vi "Main.vi"(7 "IP-Address":string, 11 "Module Admin":refnum<class "Delacor_lib_QMH_Module Admin.lvclass">) -> ()   [LabVIEW 2021, in "Safety.lvlib"]
doc: "This template is based off of the Queued Message Handler design pattern and the Queued Message Handler project template that ships with LabVIEW.\n\nThe main difference is that the queue is private to this module and communication between modules is performed via Broadcast and Request events.\n\nRequest events are wrapped in public API methods and are handled in the Event Handling Loop (EHL) of this VI. Any module can register for Broadcast events sent by this module. The EHL generates messages based on user interface actions.\n\nThe Message Handling Loop (MHL) processes messages generated by the EHL, or by other messages. The messages are string values, so new messages can be added easily to the Message Cases case structure in the MHL. Each message cluster can also provide an optional value for Message Data, which is a variant that can be converted to whatever message-specific data is required.\n_____\nBased on DQMH Project Template 7.0.1.1316."
uses:
  Safety.lvlib
  <vilib>/Delacor/Delacor QMH/Libraries/Module Admin_class/Delacor_lib_QMH_Module Admin.lvclass
  Module Data--cluster.ctl
  <vilib>/Wovalab/Utilities/Helper Loop Periodic Timing/Helper Loop Periodic Timing.lvclass/Helper Loop Periodic Timing.ctl
  <vilib>/Delacor/Delacor QMH/Libraries/Message Queue_class/Delacor_lib_QMH_Message Queue.lvclass/Delacor_lib_QMH_Message Queue.ctl
  Do Something Argument--cluster.ctl
  Do Something Else Argument--cluster.ctl
  Do Something Else and Wait for Reply Argument--cluster.ctl
  Do Something Else and Wait (Reply Payload)--cluster.ctl
  Stop Argument--cluster.ctl
  <vilib>/Delacor/Delacor QMH/Libraries/Module Admin_class/Delacor_lib_QMH_Module Admin.lvclass/Delacor_lib_QMH_Module Admin.ctl
  <vilib>/Utility/miscctls.llb/LVPointTypeDef.ctl
  <vilib>/Delacor/Delacor QMH/Libraries/Message Queue_class/Delacor_lib_QMH_Enqueue Message (Single).vi
  <vilib>/Delacor/Delacor QMH/Libraries/Module Admin_class/Delacor_lib_QMH_Get External Launch.vi
  <vilib>/Wovalab/Utilities/Helper Loop Periodic Timing/U32 Max Value--constant.vi
  <vilib>/Wovalab/Utilities/Helper Loop Periodic Timing/Update Last Execution Time.vi
  <vilib>/Wovalab/Utilities/Helper Loop Periodic Timing/Helper Loop Periodic Timing.lvclass
  <vilib>/Delacor/Delacor QMH/Libraries/Message Queue_class/Delacor_lib_QMH_Message Queue.lvclass
  <userlib>/_OpenG.lib/time/time.llb/openg_time.lvlib
panel:
  out "error out":errorcluster
  out "X":dbl
  out "Status":string
  in  "Simulate MHL Error":bool
  in  "Simulate EHL Error":bool
  in  "Do Something Else <Replace Me>":bool
  in  "Do Something <Replace Me>":bool
  # "These controls have associated \"Value Changed\" events configured in the Event Structure on the diagram.\n\nReplace them (and reconfigure the Event Structure) with the controls you need for your application. \n\nOther processes communicate with this Module via its Public API (wrappers for its Request Events).\n\nThis Module communicates with other processes via its Broadcast Events.\nAny process that wants to receive these messages can register for this module's Broadcast events."
  # "This template is for the DQMH framework. See the block diagram for more information on how to use this template."
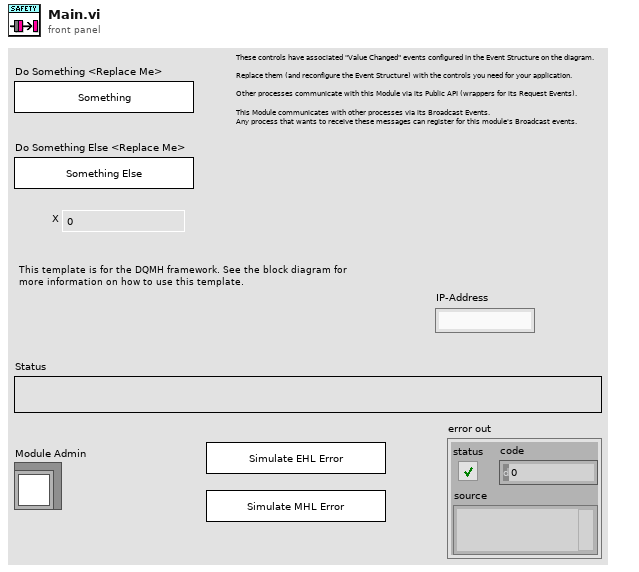
[diagram p1: front panel]
types:
  T1 = typedef "Safety.lvlib/Request Events--cluster.ctl" = cluster{"Stop Module":refnum<user-event>, "Do Something":refnum<user-event>, "Do Something Else":refnum<user-event>, "Do Something Else and Wait for Reply":refnum<user-event>, "Show Panel":refnum<user-event>, "Hide Panel":refnum<user-event>, "Get Module Execution Status":refnum<user-event>, "Show Diagram":refnum<user-event>}
  T2 = typedef "Safety.lvlib/Module Data--cluster.ctl" = cluster{"Status":string, "IP-Address":string}
  T3 = typedef "Safety.lvlib/Do Something Argument--cluster.ctl" = cluster{"Do Something Msg":string}
  T4 = typedef "Safety.lvlib/Do Something Else Argument--cluster.ctl" = cluster{"Do Something Else Msg":string, "X":dbl}
  T5 = typedef "Safety.lvlib/Do Something Else and Wait for Reply Argument--cluster.ctl" = cluster{"Do Something Else Msg":string, "X":dbl, "Wait Notifier":refnum<notifier>, "wait for reply":bool}
  T6 = enum32{"invalid lock state", "Not Locked", "Locked (No Password)", "Password-protected"}
  T7 = typedef "Safety.lvlib/Stop Argument--cluster.ctl" = cluster{"Origin":string, "Exit via Stop Module Req?":bool, "Wait for Module to stop?":bool}
  T8 = typedef "LVPointTypeDef.ctl" = cluster{"Horizontal":i16, "Vertical":i16}
  T9 = enum32{"Invalid", "Standard", "Closed", "Hidden", "Minimized", "Maximized"}
  T10 = typedef "Safety.lvlib/Do Something Else and Wait (Reply Payload)--cluster.ctl" = cluster{"Value":dbl, "error":errorcluster}
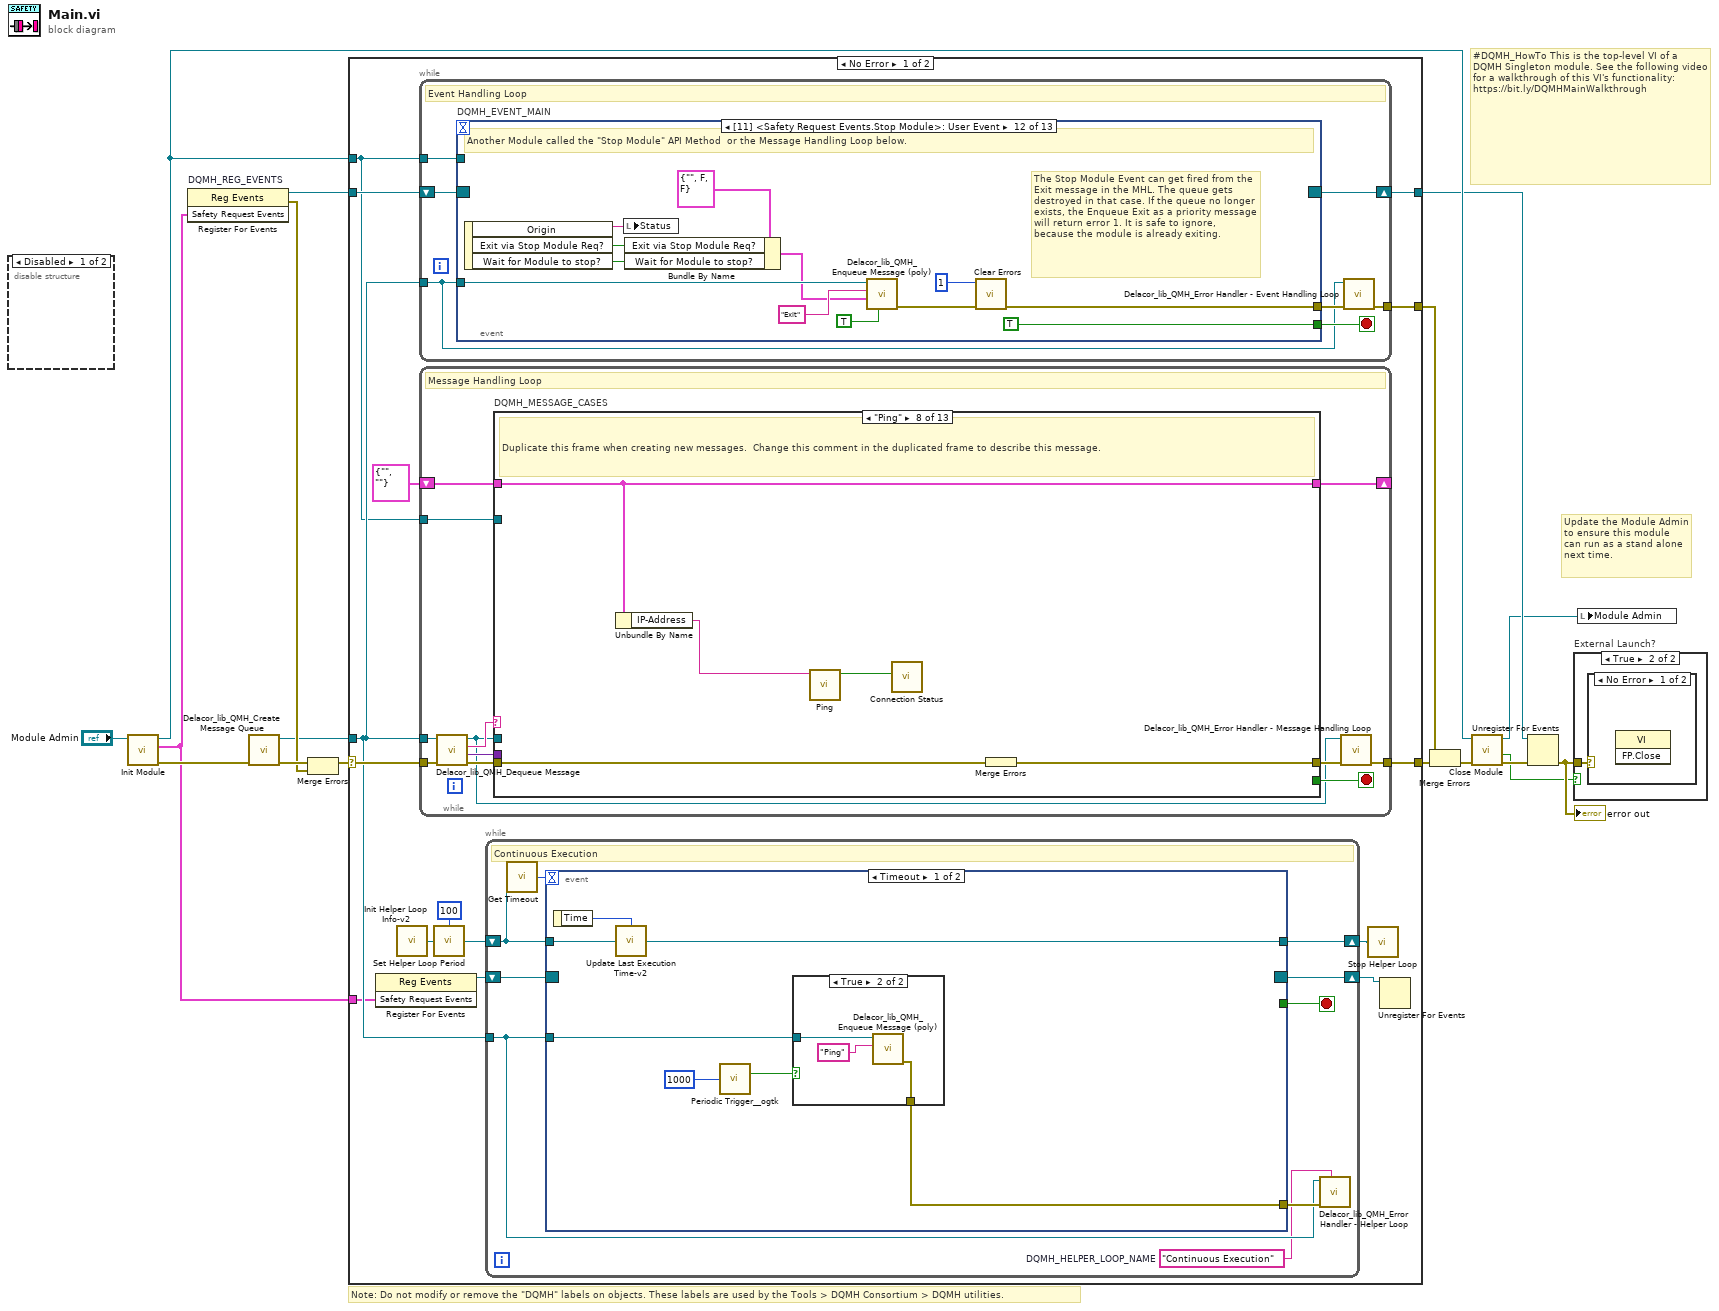
[diagram p0: block diagram]
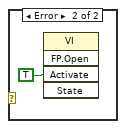
[diagram p4: hidden frame]
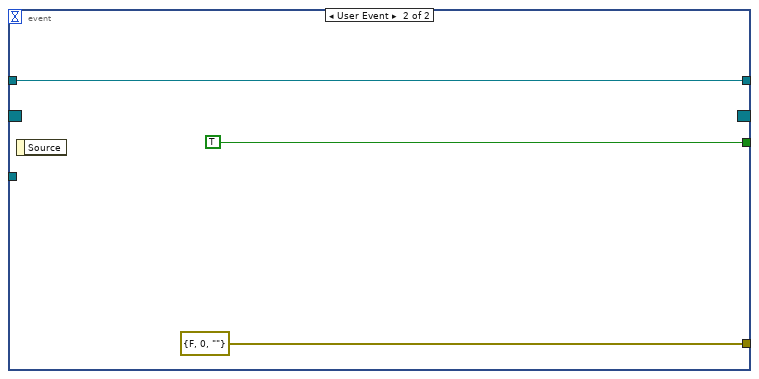
[diagram p6: hidden frame]
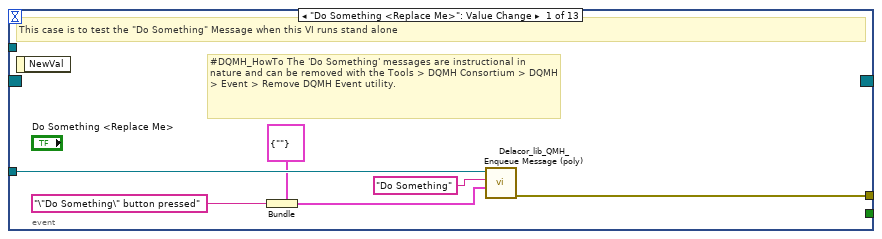
[diagram p7: hidden frame]
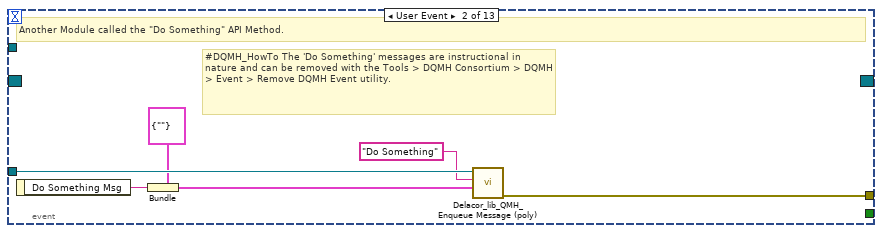
[diagram p8: hidden frame]
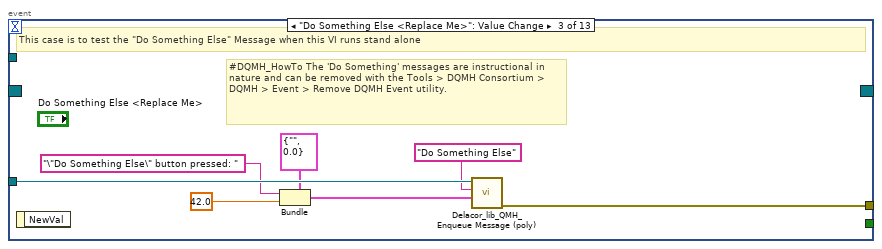
[diagram p9: hidden frame]
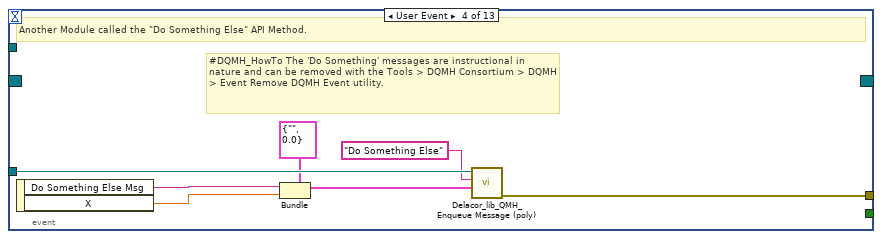
[diagram p10: hidden frame]
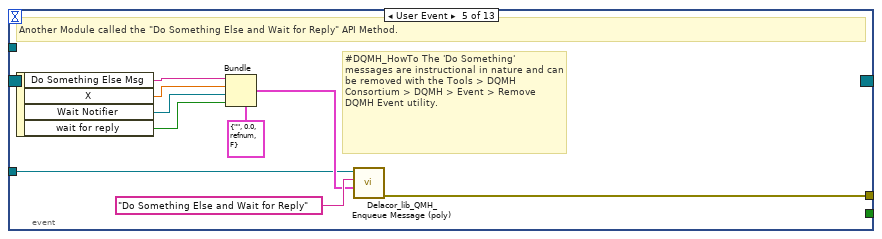
[diagram p11: hidden frame]
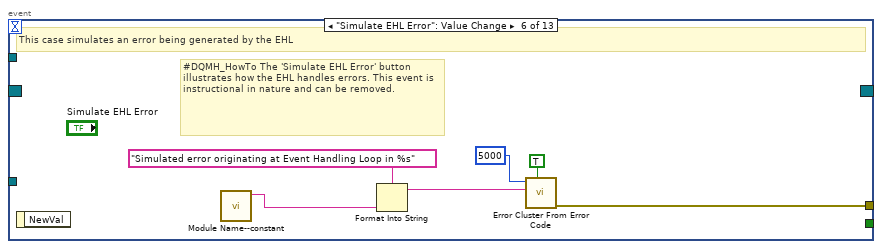
[diagram p12: hidden frame]
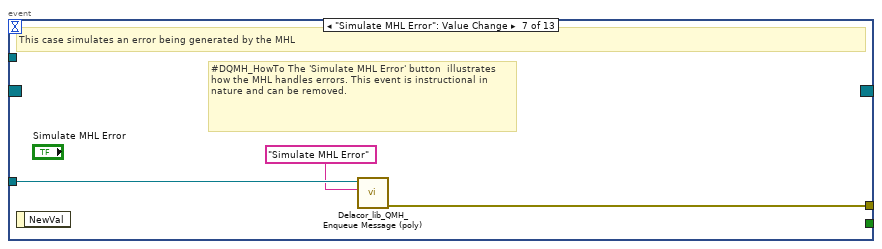
[diagram p13: hidden frame]
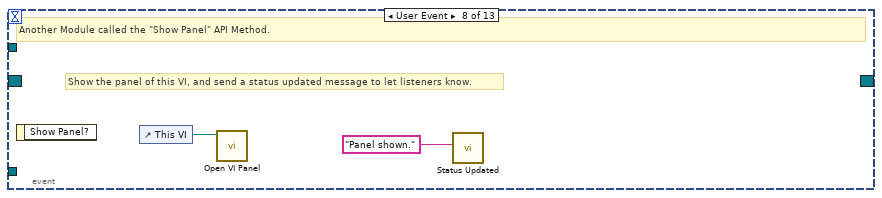
[diagram p14: hidden frame]
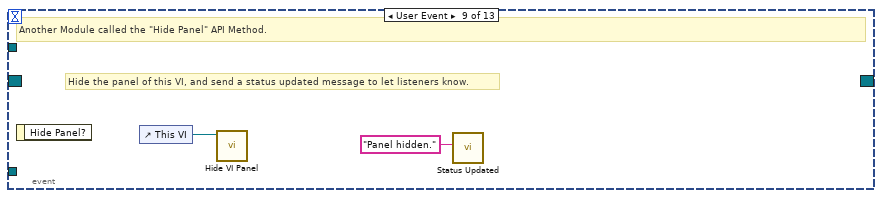
[diagram p15: hidden frame]
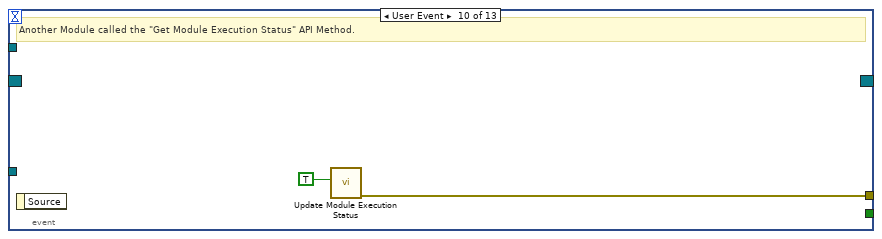
[diagram p16: hidden frame]
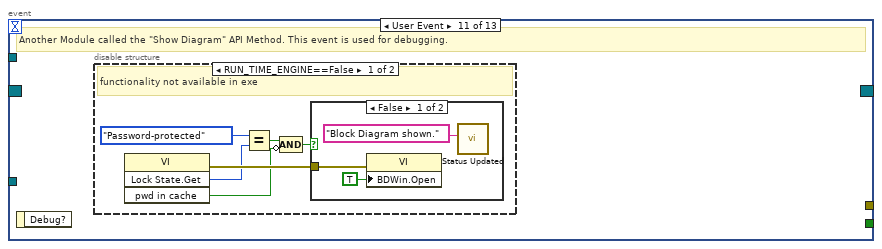
[diagram p17: hidden frame]
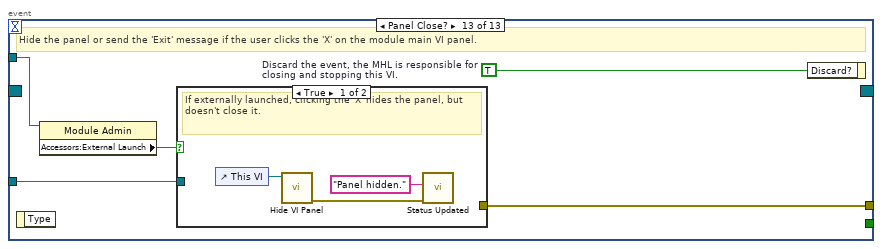
[diagram p20: hidden frame]
diagram:
  # "#DQMH_HowTo This is the top-level VI of a DQMH Singleton module. See the following video for a walkthrough of this VI's functionality: https://bit.ly/DQMHMainWalkthrough"
  # "Note: Do not modify or remove the \"DQMH\" labels on objects. These labels are used by the Tools > DQMH Consortium > DQMH utilities."
  # "Update the Module Admin to ensure this module can run as a stand alone next time."
  n1 = disable-structure shown="Disabled" {
    frame Disabled {
    }
    frame Enabled {
    }
  }
  n2 = call "Init Module.vi"("Singleton Module Admin in"="Module Admin") -> ("error out"=w16:errorcluster, "Safety Request Events"=w1:T1, "Singleton Module Admin out"=w8:refnum<class "Delacor_lib_QMH_Module Admin.lvclass">)  [unwired: 8 in]
  n3 = register-events "DQMH_REG_EVENTS"(w1) -> (reference out=w6:refnum<event-registration>, error out=w9:errorcluster)  [unwired: 2 in]
  n4 = call <vilib>:"Delacor_lib_QMH_Create Message Queue.vi"("error in"=w16) -> ("error out"=w11:errorcluster, "Message Queue"=w5:refnum<class "Delacor_lib_QMH_Message Queue.lvclass">)  [unwired: 9 in]
  n5 = Merge Errors(w11, w9) -> (w10:errorcluster)
  n6 = case shown="No Error" w10 {
    selector: w10 -> [w30 w301]
    tunnel: [w32 w300] -> w17
    tunnel: [w29 w299] -> w7
    tunnel: w6 -> [w27 w299]
    tunnel: w5 -> [w26 w294]
    tunnel: [w31 _] -> w14
    tunnel: w8 -> [w25 w295]
    tunnel: w1 -> [w24 _]
    frame No Error {
      n7 = register-events ("DQMH_HELPER_REGFOREVENTS")(w24) -> (reference out=w22:refnum<event-registration>)  [unwired: 2 in, 1 out]
      n8 = call <vilib>:"Init Helper Loop Info-v2.vi"() -> ("Helper Loop Periodic Timing"=w20:refnum<class "Helper Loop Periodic Timing.lvclass">)  [unwired: 1 in]
      n9 = while {
        tunnel: w26 -> [w55]
        shift-right: [w58] -> w29
        shift-left: w27 -> [w59]
        tunnel: [w60] -> w31
        tunnel: w25 -> [w56]
        stop <- w57 stop-if-true
        # "Event Handling Loop"
        n10 = event "DQMH_EVENT_MAIN" shown="[11] <Safety Request Events.Stop Module>: User Event" {
          selector: w59 -> [_ _ _ _ _ _ _ _ _ _ _ _ _]
          dyn-events: [_ _ _ _ _ _ _ _ _ _ _ _ _] -> w58
          timeout: _ -> [_ _ _ _ _ _ _ _ _ _ _ _ _]
          tunnel: [_ _ _ _ _ _ _ _ _ _ _ TRUE ("Discard?") _] -> w57
          tunnel: w55 -> [w66 w72 w79 w86 w89 _ w104 _ _ _ _ w128 w135]
          tunnel: [w67 w73 w80 w87 w96 w102 w105 _ _ w111 _ w131 w137] -> w61
          tunnel: w56 -> [_ _ _ _ _ _ _ _ _ _ _ _ w134]
          event "Do Something <Replace Me>": Value Change {
            # "#DQMH_HowTo The 'Do Something' messages are instructional in nature and can be removed with the Tools > DQMH Consortium > DQMH > Event > Remove DQMH Event utility."
            # "This case is to test the \"Do Something\" Message when this VI runs stand alone"
            n11 = event-data() -> ()  [unwired: 1 in, 1 out]
            n12 = Bundle(cluster=T3 {"Do Something Msg"=""} ("Do Something Argument"), "Do Something Msg"="\"Do Something\" button pressed" ("\"Do Something\" button pressed")) -> (w62:T3)
            n13 = call-poly <vilib>:"Delacor_lib_QMH_Enqueue Message (poly).vi"("Message Data"=w62, "Message"="Do Something", "Message Queue in"=w66) -> ("error out"=w67:errorcluster)  [unwired: 7 in, 1 out]
          }
          event User Event {
            # "#DQMH_HowTo The 'Do Something' messages are instructional in nature and can be removed with the Tools > DQMH Consortium > DQMH > Event > Remove DQMH Event utility."
            # "Another Module called the \"Do Something\" API Method."
            n14 = event-data() -> ("Do Something Msg"=w69:string)  [unwired: 1 in]
            n15 = Bundle(cluster=T3 {"Do Something Msg"=""} ("Do Something Argument"), "Do Something Msg"=w69) -> (w68:T3)
            n16 = call-poly <vilib>:"Delacor_lib_QMH_Enqueue Message (poly).vi"("Message Data"=w68, "Message"="Do Something", "Message Queue in"=w72) -> ("error out"=w73:errorcluster)  [unwired: 7 in, 1 out]
          }
          event "Do Something Else <Replace Me>": Value Change {
            # "#DQMH_HowTo The 'Do Something' messages are instructional in nature and can be removed with the Tools > DQMH Consortium > DQMH > Event > Remove DQMH Event utility."
            # "This case is to test the \"Do Something Else\" Message when this VI runs stand alone"
            n17 = event-data() -> ()  [unwired: 1 in, 1 out]
            n18 = Bundle(cluster=T4 {"Do Something Else Msg"="", "X"=0.0} ("Do Something Else Argument"), "Do Something Else Msg"="\"Do Something Else\" button pressed: " ("\"Do Something Else\" button pressed"), "X"=42.0) -> (w76:T4)
            n19 = call-poly <vilib>:"Delacor_lib_QMH_Enqueue Message (poly).vi"("Message Data"=w76, "Message"="Do Something Else", "Message Queue in"=w79) -> ("error out"=w80:errorcluster)  [unwired: 7 in, 1 out]
          }
          event User Event {
            # "#DQMH_HowTo The 'Do Something' messages are instructional in nature and can be removed with the Tools > DQMH Consortium > DQMH > Event Remove DQMH Event utility."
            # "Another Module called the \"Do Something Else\" API Method."
            n20 = event-data() -> ("Do Something Else Msg"=w82:string, "X"=w81:dbl)  [unwired: 1 in]
            n21 = Bundle(cluster=T4 {"Do Something Else Msg"="", "X"=0.0} ("Do Something Else Argument"), "Do Something Else Msg"=w82, "X"=w81) -> (w83:T4)
            n22 = call-poly <vilib>:"Delacor_lib_QMH_Enqueue Message (poly).vi"("Message Data"=w83, "Message"="Do Something Else", "Message Queue in"=w86) -> ("error out"=w87:errorcluster)  [unwired: 7 in, 1 out]
          }
          event User Event {
            # "#DQMH_HowTo The 'Do Something' messages are instructional in nature and can be removed with the Tools > DQMH Consortium > DQMH > Event > Remove DQMH Event utility."
            # "Another Module called the \"Do Something Else and Wait for Reply\" API Method."
            n23 = event-data() -> ("Do Something Else Msg"=w92:string, "X"=w91:dbl, "Wait Notifier"=w90:refnum<notifier>, "wait for reply"=w88:bool)  [unwired: 1 in]
            n24 = Bundle(cluster=T5 {"Do Something Else Msg"="", "X"=0.0, "Wait Notifier"=refnum, "wait for reply"=FALSE} ("Do Something Else and Wait for Reply Argument"), "Do Something Else Msg"=w92, "X"=w91, "Wait Notifier"=w90, "wait for reply"=w88) -> (w93:T5)
            n25 = call-poly <vilib>:"Delacor_lib_QMH_Enqueue Message (poly).vi"("Message Data"=w93, "Message"="Do Something Else and Wait for Reply", "Message Queue in"=w89) -> ("error out"=w96:errorcluster)  [unwired: 7 in, 1 out]
          }
          event "Simulate EHL Error": Value Change {
            # "#DQMH_HowTo The 'Simulate EHL Error' button  illustrates how the EHL handles errors. This event is instructional in nature and can be removed."
            # "This case simulates an error being generated by the EHL"
            n26 = event-data() -> ()  [unwired: 1 in, 1 out]
            n27 = call "Module Name--constant.vi"() -> ("Module Name"=w99:string)  [unwired: 11 in]
            n28 = Format Into String(format string="Simulated error originating at Event Handling Loop in %s", w99) -> (resulting string=w100:string)  [unwired: 2 in, 1 out]
            n29 = call <vilib>:"Error Cluster From Error Code.vi"("show call chain? (False)"=TRUE, "error message (\"\")"=w100, "error code (0)"=5000) -> ("error out"=w102:errorcluster)  [unwired: 6 in]
          }
          event "Simulate MHL Error": Value Change {
            # "#DQMH_HowTo The 'Simulate MHL Error' button  illustrates how the MHL handles errors. This event is instructional in nature and can be removed."
            # "This case simulates an error being generated by the MHL"
            n30 = event-data() -> ()  [unwired: 1 in, 1 out]
            n31 = call-poly <vilib>:"Delacor_lib_QMH_Enqueue Message (poly).vi"("Message"="Simulate MHL Error", "Message Queue in"=w104) -> ("error out"=w105:errorcluster)  [unwired: 8 in, 1 out]
          }
          event User Event {
            # "Show the panel of this VI, and send a status updated message to let listeners know."
            # "Another Module called the \"Show Panel\" API Method."
            n32 = event-data() -> ()  [unwired: 1 in, 1 out]
            n33 = control-ref of="This VI"() -> (w107:refnum<vi>)
            n34 = call "Open VI Panel.vi"("VI"=w107) -> ()  [unwired: 10 in, 1 out]
            n35 = call "Status Updated.vi"("Status"="Panel shown." ("format string")) -> ()  [unwired: 10 in, 1 out]
          }
          event User Event {
            # "Hide the panel of this VI, and send a status updated message to let listeners know."
            # "Another Module called the \"Hide Panel\" API Method."
            n36 = event-data() -> ()  [unwired: 1 in, 1 out]
            n37 = control-ref of="This VI"() -> (w109:refnum<vi>)
            n38 = call "Hide VI Panel.vi"("VI"=w109) -> ()  [unwired: 10 in, 1 out]
            n39 = call "Status Updated.vi"("Status"="Panel hidden." ("format string")) -> ()  [unwired: 10 in, 1 out]
          }
          event User Event {
            # "Another Module called the \"Get Module Execution Status\" API Method."
            n40 = event-data() -> ()  [unwired: 1 in, 1 out]
            n41 = call "Update Module Execution Status.vi"("Running?"=TRUE) -> ("error out"=w111:errorcluster)  [unwired: 10 in]
          }
          event User Event {
            # "Another Module called the \"Show Diagram\" API Method. This event is used for debugging."
            n42 = event-data() -> ()  [unwired: 1 in, 1 out]
            n43 = disable-structure shown="RUN_TIME_ENGINE==False" {
              frame condition #0 (active) {
                # "functionality not available in exe"
                n44 = invoke on="Invoke Node" class="VI" method="Lock State.Get"() -> (error out=w117:errorcluster, "Get Lock State"=w116:T6, "pwd in cache"=w113:bool)  [unwired: 4 in, 1 out]
                n45 = Equal?(x=T6."Password-protected", y=w116) -> (x = y?=w114:bool)
                n46 = Compound Arithmetic op=AND(w114, invert w113) -> (w112:bool)
                n47 = case shown="False" w112 {
                  tunnel: w117 -> [w120 _]
                  frame False {
                    n48 = property on="Property Node" class="VI"(error in=w120, "BDWin.Open"=TRUE ("Block Diagram Window:Open")) -> ()  [unwired: 1 in, 2 out]
                    n49 = call "Status Updated.vi"("Status"="Block Diagram shown." ("format string")) -> ()  [unwired: 10 in, 1 out]
                  }
                  frame True {
                    # "Password-protected VI, and the password is not in the cache. Do not show the diagram."
                  }
                }
              }
              frame condition #1 {
              }
            }
          }
          event User Event {
            # "The Stop Module Event can get fired from the Exit message in the MHL. The queue gets destroyed in that case. If the queue no longer exists, the Enqueue Exit as a priority message will return error 1. It is safe to ignore, because the module is already exiting."
            # "Another Module called the \"Stop Module\" API Method  or the Message Handling Loop below."
            n50 = event-data() -> ("Origin"=w127:string, "Exit via Stop Module Req?"=w123:bool, "Wait for Module to stop?"=w122:bool)  [unwired: 1 in]
            n51 = local write "Status"(w127) -> ()
            n52 = Bundle By Name(cluster=T7 {"Origin"="", "Exit via Stop Module Req?"=FALSE, "Wait for Module to stop?"=FALSE} ("Stop Argument"), "Exit via Stop Module Req?"=w123, "Wait for Module to stop?"=w122) -> (w121:T7)
            n53 = call-poly <vilib>:"Delacor_lib_QMH_Enqueue Message (poly).vi"("Priority Message? (F)"=TRUE, "Message Data"=w121, "Message"="Exit", "Message Queue in"=w128) -> ("error out"=w132:errorcluster)  [unwired: 6 in, 1 out]
            n54 = call <vilib>:"Clear Errors.vi"("error in (no error)"=w132, "specific error code to clear (0: all)"=1) -> ("error out"=w131:errorcluster)  [unwired: 4 in, 1 out]
          }
          event Panel Close? {
            w136 = TRUE  # Discard the event, the MHL is responsible for closing and stopping this VI.
            # "Hide the panel or send the 'Exit' message if the user clicks the 'X' on the module main VI panel."
            n55 = event-data() -> ()  [unwired: 1 in, 1 out]
            n56 = property on="Property Node" class="Module Admin"(reference=w134) -> ("Accessors:External Launch"=w133:bool)  [unwired: 1 in, 2 out]
            n57 = case shown="True" w133 {
              tunnel: w135 -> [_ w143]
              tunnel: [_ w144] -> w137
              frame True {
                # "If externally launched, clicking the 'X' hides the panel, but doesn't close it."
                n58 = control-ref of="This VI"() -> (w140:refnum<vi>)
                n59 = call "Hide VI Panel.vi"("VI"=w140) -> ("error out"=w138:errorcluster)  [unwired: 10 in]
                n60 = call "Status Updated.vi"("error in"=w138, "Status"="Panel hidden." ("format string")) -> ()  [unwired: 9 in, 1 out]
              }
              frame False {
                # "If run as a stand-alone VI, clicking the panel 'X' stops the VI."
                n61 = call-poly <vilib>:"Delacor_lib_QMH_Enqueue Message (poly).vi"("Priority Message? (F)"=TRUE, "Message"="Exit", "Message Queue in"=w143) -> ("error out"=w144:errorcluster)  [unwired: 7 in, 1 out]
              }
            }
            n62 = event-data ("Event Filter Node")("Discard?"=w136) -> ()  [unwired: 1 in, 1 out]
          }
        }
        n63 = call-dynamic "Delacor_lib_QMH_Error Handler - Event Handling Loop.vi"("error in"=w61, "Message Queue in"=w55) -> ("dup error in"=w60:errorcluster)  [unwired: 8 in, 1 out]
      }
      n64 = while {
        tunnel: w26 -> [w145]
        shift-right: [w153] -> _
        shift-left: T2 {"Status"="", "IP-Address"=""} ("Data Cluster") -> [w154]
        tunnel: w30 -> [w156]
        tunnel: [w148] -> w32
        tunnel: w25 -> [w149]
        stop <- w152 stop-if-true
        # "Message Handling Loop"
        n65 = call-dynamic "Delacor_lib_QMH_Dequeue Message.vi"("error in"=w156, "Message Queue in"=w145) -> ("error out"=w155:errorcluster, "Message Data"=w150:variant, "Message"=w151:string, "Message Queue out"=w146:refnum<class "Delacor_lib_QMH_Message Queue.lvclass">)  [unwired: 6 in]
        n66 = case "DQMH_MESSAGE_CASES" shown="\"Ping\"" w151 {
          selector: w151 -> [_ _ _ _ _ _ _ _ _ _ _ _ w289]
          tunnel: w146 -> [w158 _ _ _ _ _ _ _ _ _ w255 w277 _]
          tunnel: w155 -> [w177 w184 w186 w194 w203 w222 w235 w240 w242 w251 w262 w283 w292]
          tunnel: [w159 w183 w186 w192 w202 w221 w234 w239 w242 w250 w258 w278 w293] -> w147
          tunnel: w154 -> [w167 w182 w185 w191 w201 w218 w233 w238 w241 w248 w257 w276 w290]
          tunnel: [w166 w181 w185 w191 w201 w218 w233 w238 w241 w248 w257 w276 w290] -> w153
          tunnel: [_ _ _ _ _ _ _ _ _ _ _ w275 _] -> w152
          tunnel: w150 -> [_ _ _ w190 w198 w215 _ _ _ _ w256 w274 _]
          tunnel: w149 -> [w168 _ _ _ _ _ _ _ _ _ w254 w269 _]
          frame "Initialize" {
            w162 = "Initial Message" ("Initial Message")
            # "#CodeNeeded - Initialize the appearance of the front panel."
            # "#CodeNeeded - Initialize your state data here."
            # "Initialize - Any operation that needs to be done before the module can receive messages. Synchronize Caller Events.vi will inform Start Module.vi that the module has launched and is ready to receive messages. Module Did Init.vi will broadcast that the module initialized."
            n67 = call "Synchronize Caller Events.vi"("error in"=w177, "Singleton Module Admin in"=w168) -> ("error out"=w176:errorcluster, "Singleton Module Admin out"=w163:refnum<class "Delacor_lib_QMH_Module Admin.lvclass">)  [unwired: 8 in]
            n68 = property on="Property Node" class="Module Admin"(reference=w163) -> ("Accessors:External Launch"=w172:bool)  [unwired: 1 in, 2 out]
            n69 = Select(t=T9."Hidden" ("State"), s=w172, f=T9."Standard" ("State")) -> (s? t:f=w169:T9)
            n70 = call "Module Name--constant.vi"() -> ("Module Name"=w175:string)  [unwired: 11 in]
            n71 = property on="Property Node" class="VI"("Front Panel.Title"=w175) -> (reference out=w174:refnum<vi>, error out=w179:errorcluster)  [unwired: 2 in]
            n72 = call "Module Name--constant.vi"() -> ("Module Name"=w164:string)  [unwired: 11 in]
            n73 = invoke on="Invoke Node" class="VI" method="FP.Open"(reference=w174, error in=w179, "State"=w169) -> (reference out=w173:refnum<vi>, error out=w178:errorcluster)  [unwired: 2 in, 3 out]
            n74 = Bundle By Name(cluster=w167, "Status"=w162) -> (w166:T2)
            n75 = call "Module Did Init.vi"("error in"=w176, "Initialized?"=TRUE, "Origin"=w164) -> ("error out"=w160:errorcluster)  [unwired: 8 in]
            n76 = invoke on="Invoke Node" class="VI" method="FP.Center"(reference=w173, error in=w178) -> ()  [unwired: 1 in, 3 out]
            n77 = property on="Pane" class="Pane"("Origin"=T8 {"Horizontal"=0, "Vertical"=0}) -> ()  [unwired: 2 in, 2 out]
            n78 = call-poly <vilib>:"Delacor_lib_QMH_Enqueue Message (poly).vi"("error in"=w160, "Message"="Init-1", "Message Queue in"=w158) -> ("error out"=w159:errorcluster)  [unwired: 7 in, 1 out]
            "Status" <- w162
          }
          frame "Init-1" {
            # "Duplicate this frame when creating new messages.  Change this comment in the duplicated frame to describe this message."
            n79 = Bundle By Name(cluster=w182, "IP-Address"="IP-Address") -> (w181:T2)
            n80 = Merge Errors(w184) -> (w183:errorcluster)
          }
          frame "---Module Specific---" {
            # "Separator -- The following cases handle messages specific to this Module."
          }
          frame "Do Something" {
            # "#DQMH_HowTo The 'Do Something' messages are instructional in nature and can be removed with the Tools > DQMH Consortium > DQMH > Event > Remove DQMH Event utility."
            # "Do Something - Replace this message with functionality for your own application. Note that this message also fires the \"Did Something\" broadcast event."
            n81 = Variant To Data(error in=w194, type=T3 {"Do Something Msg"=""} ("Do Something Argument"), Variant=w190) -> (data=w189:T3, error out=w193:errorcluster)
            n82 = Unbundle By Name(w189) -> ("Do Something Msg"=w187:string)
            n83 = call "Did Something.vi"("error in"=w193, "Did Something Msg"=w187) -> ("error out"=w192:errorcluster)  [unwired: 9 in]
            n84 = local write "Status"(w187) -> ()
            n85 = call "Status Updated.vi"("Status"=w187) -> ()  [unwired: 10 in, 1 out]
          }
          frame "Do Something Else" {
            # "#DQMH_HowTo The 'Do Something' messages are instructional in nature and can be removed with the Tools > DQMH Consortium > DQMH > Event > Remove DQMH Event utility."
            # "Do Something Else - Replace this message with functionality for your own application."
            n86 = Variant To Data(error in=w203, type=T4 {"Do Something Else Msg"="", "X"=0.0} ("Do Something Else Argument"), Variant=w198) -> (data=w199:T4, error out=w202:errorcluster)
            n87 = Unbundle By Name(w199) -> ("Do Something Else Msg"=w197:string, "X"=w196:dbl)
            "X" <- w196
            n88 = Format Into String(initial string=w197, w196) -> (resulting string=w195:string)  [unwired: 2 in, 1 out]
            n89 = local write "Status"(w195) -> ()
            n90 = call "Status Updated.vi"("Status"=w195) -> ()  [unwired: 10 in, 1 out]
          }
          frame "Do Something Else and Wait for Reply" {
            w210 = "X(%.2f)+Offset(%.2f)=%.2f"  # status message format string
            # "#DQMH_HowTo The 'Do Something' messages are instructional in nature and can be removed."
            # "Send back X with a random offset"
            # "Do Something Else and Wait for Reply - Replace this message with functionality for your own application. Note that this message must fire a notifier to let callers know it has finished execution, and it returns an error if the 'Value' is negative."
            n91 = Variant To Data(error in=w222, type=T5 {"Do Something Else Msg"="", "X"=0.0, "Wait Notifier"=refnum, "wait for reply"=FALSE} ("Do Something Else and Wait for Reply Argument"), Variant=w215) -> (data=w216:T5, error out=w220:errorcluster)
            n92 = Unbundle By Name(w216) -> ("Wait Notifier"=w204:refnum<notifier>, "Do Something Else Msg"=w214:string, "X"=w211:dbl, "wait for reply"=w207:bool)
            n93 = Random Number (0-1)() -> (number: 0 to 1=w212:dbl)
            n94 = Add(x=w212, y=w211) -> (x+y=w206:dbl)
            n95 = Less Than 0?(x=w206) -> (x < 0?=w209:bool)
            n96 = local write "X"(w211) -> ()
            n97 = case shown="True" w209 {
              tunnel: [_ w232] -> w219
              frame False {
              }
              frame True {
                n98 = call <vilib>:"Error Cluster From Error Code.vi"("show call chain? (False)"=TRUE, "error message (\"\")"="The 'Something Else and Wait for Reply' message generated a negative number, which is considered an error condition.", "error code (0)"=5000) -> ("error out"=w232:errorcluster)  [unwired: 6 in]
              }
            }
            n99 = Format Into String(format string=w210, initial string=w214, w211, w212, w206) -> (resulting string=w208:string)  [unwired: 1 in, 1 out]
            n100 = Bundle By Name(cluster=T10 {"Value"=0.0, "error"={"status"=FALSE, "code"=0, "source"=""}} ("notification"), "error"=w219, "Value"=w206) -> (w205:T10)
            n101 = local write "Status"(w208) -> ()
            n102 = call "Status Updated.vi"("Status"=w208) -> ()  [unwired: 10 in, 1 out]
            n103 = case shown="True" w207 {
              tunnel: w205 -> [_ w225]
              tunnel: w204 -> [_ w224]
              frame False {
              }
              frame True {
                # "Simulate an operation that requires a wait."
                n104 = flat-sequence {
                  tunnel: w225 -> [w228]
                  tunnel: w224 -> [w227]
                  tunnel: w223 -> [_]
                  frame #0 {
                    n105 = Send Notification(notification=w228, notifier=w227) -> ()  [unwired: 1 in, 2 out]
                  }
                }
                n106 = Wait (ms)(milliseconds to wait=u32 1000) -> (millisecond timer value=w223:u32)
              }
            }
            n107 = Merge Errors(w220, w219) -> (w221:errorcluster)
          }
          frame "---Copy This Frame---" {
            # "Duplicate this frame when creating new messages.  Change this comment in the duplicated frame to describe this message."
            n108 = Merge Errors(w235) -> (w234:errorcluster)
          }
          frame "Ping" {
            # "Duplicate this frame when creating new messages.  Change this comment in the duplicated frame to describe this message."
            n109 = Unbundle By Name(w238) -> ("IP-Address"=w237:string)
            n110 = call "Ping.vi"("hostNameOrAddress"=w237) -> ("Ping Status"=w236:bool)  [unwired: 9 in, 1 out]
            n111 = call "Connection Status.vi"("Connection Status"=w236) -> ()  [unwired: 10 in, 1 out]
            n112 = Merge Errors(w240) -> (w239:errorcluster)
          }
          frame "---Exit and Error Handling---" {
            # "Separator - The following cases handle errors and exit messages."
          }
          frame "Simulate MHL Error" {
            # "#DQMH_HowTo The 'Simulate MHL Error' button  illustrates how the MHL handles errors. This event is instructional in nature and can be removed."
            # "Simulate an error occurring at the MHL"
            n113 = call "Module Name--constant.vi"() -> ("Module Name"=w244:string)  [unwired: 11 in]
            n114 = Format Into String(format string="Simulated error originating at Message Handling Loop in %s", w244) -> (resulting string=w245:string)  [unwired: 2 in, 1 out]
            n115 = call <vilib>:"Error Cluster From Error Code.vi"("show call chain? (False)"=TRUE, "error message (\"\")"=w245, "error code (0)"=5001) -> ("error out"=w249:errorcluster)  [unwired: 6 in]
            n116 = Merge Errors(w251, w249) -> (w250:errorcluster)
          }
          frame "Error" {
            # "#CodeRecommended - If the module is running in standalone mode (External Launch = FALSE), this code will pop up an error dialog and call the 'Exit' message if an error occurs. Add more fine-grained error management here."
            # "Error - Check the error message data and respond accordingly. This message is sent by the \"Error Handler\" VIs at the end of each loop in this application."
            n117 = property on="Property Node" class="Module Admin"(reference=w254) -> ("Accessors:External Launch"=w253:bool)  [unwired: 1 in, 2 out]
            n118 = Variant To Data(error in=w262, type=errorcluster {"status"=FALSE, "code"=0, "source"=""} ("error constant"), Variant=w256) -> (data=w252:errorcluster, error out=w260:errorcluster)
            n119 = local write "error out"(w252) -> ()
            n120 = call "Error Reported.vi"("Error"=w252) -> ()  [unwired: 10 in, 1 out]
            n121 = case shown="False" w253 {
              tunnel: [w267 _] -> w259
              tunnel: w255 -> [w265 _]
              tunnel: w252 -> [w266 _]
              frame False {
                n122 = disable-structure shown="Default" {
                  disable-tunnel: w266 -> [w268 _]
                  frame condition #0 (active) {
                    # "If the module is running standalone, then pop up an error dialog and call the \"Exit\" message."
                    n123 = call <vilib>:"Simple Error Handler.vi"("error in (no error)"=w268) -> ()  [unwired: 4 in, 5 out]
                  }
                  frame condition #1 {
                    # "To prevent the Simple Error Handler VI from being loaded (e.g. when deploying to a Real-Time target), add the Conditional Disable Symbol \"DQMH_Disable_SEH\" to your project and set it to TRUE."
                  }
                }
                n124 = call-poly <vilib>:"Delacor_lib_QMH_Enqueue Message (poly).vi"("Priority Message? (F)"=TRUE, "Message"="Exit", "Message Queue in"=w265) -> ("error out"=w267:errorcluster)  [unwired: 7 in, 1 out]
              }
              frame True {
                # "If the module was launched externally, calling the Error Reported broadcast VI is the only action performed by the \"Error\" message. The module's caller can then process the error appropriately."
              }
            }
            n125 = Merge Errors(w260, w259) -> (w258:errorcluster)
          }
          frame "Exit" {
            w273 = 91  # 91: not all Exit messages will have an argument
            w275 = TRUE  # Stop the VI
            # "Release the message queue reference"
            # "#CodeNeeded - Add any required cleanup code here."
            # "Exit - Exit the application."
            n126 = Variant To Data(error in=w283, type=T7 {"Origin"="", "Exit via Stop Module Req?"=FALSE, "Wait for Module to stop?"=FALSE} ("Stop Argument"), Variant=w274) -> (data=w271:T7, error out=w280:errorcluster)
            n127 = call <vilib>:"Clear Errors.vi"("error in (no error)"=w280, "specific error code to clear (0: all)"=w273) -> ("error out"=w282:errorcluster)  [unwired: 4 in, 1 out]
            n128 = control-ref of="This VI"() -> (w270:refnum<vi>)
            n129 = call-dynamic "Delacor_lib_QMH_Release Message Queue.vi"("error in"=w282, "Message Queue"=w277) -> ("error out"=w281:errorcluster)  [unwired: 9 in]
            n130 = call "Handle Exit.vi"("Stop Argument"=w271, "Admin in"=w269, "VI reference"=w270) -> ("error out"=w279:errorcluster)  [unwired: 7 in, 1 out]
            n131 = Merge Errors(w281, w279) -> (w278:errorcluster)
            n132 = call "Error Reported.vi"("Error"=w278) -> ()  [unwired: 10 in, 1 out]
          }
          frame Default {
            # "'Default' case only runs if there is a message that isn't defined in any of the other cases.  Output a programming error."
            n133 = call "Module Name--constant.vi"() -> ("Module Name"=w288:string)  [unwired: 11 in]
            n134 = Format Into String(format string="The invalid message string \"%s\" was received in the Message Handling Loop for module \"%s\".", w289, w288) -> (resulting string=w284:string)  [unwired: 2 in, 1 out]
            n135 = call <vilib>:"Error Cluster From Error Code.vi"("show call chain? (False)"=TRUE, "error message (\"\")"=w284, "error code (0)"=1) -> ("error out"=w291:errorcluster)  [unwired: 6 in]
            n136 = Merge Errors(w292, w291) -> (w293:errorcluster)
          }
        }
        n137 = call-dynamic "Delacor_lib_QMH_Error Handler - Message Handling Loop.vi"("error in"=w147, "Message Queue in"=w146) -> ("dup error in"=w148:errorcluster)  [unwired: 8 in, 1 out]
      }
      n138 = call <vilib>:"Set Helper Loop Period.vi"("Period (ms)"=100, "Helper Loop Periodic Timing in"=w20) -> ("Helper Loop Periodic Timing out"=w21:refnum<class "Helper Loop Periodic Timing.lvclass">)  [unwired: 13 in]
      n139 = while "DQMH_HELPER_LOOP" {
        shift-right: [w41] -> w18
        shift-left: w21 -> [w34]
        shift-right: [w39] -> w23
        shift-left: w22 -> [w40]
        tunnel: w26 -> [w36]
        stop <- w38 stop-if-true
        w35 = "Continuous Execution"  # DQMH_HELPER_LOOP_NAME
        # "Continuous Execution"
        n140 = call <vilib>:"Get Timeout.vi"("Helper Loop Periodic Timing"=w34) -> ("Timeout (ms)"=w33:i32)  [unwired: 12 in, 2 out]
        n141 = event "DQMH_HELPER_EVENT_STRUCTURE" shown="[0] Timeout" {
          selector: w40 -> [_ _]
          dyn-events: [_ _] -> w39
          timeout: w33 -> [_ _]
          tunnel: w34 -> [w47 w54]
          tunnel: [w46 w54] -> w41
          tunnel: [_ TRUE] -> w38
          tunnel: [w44 errorcluster {"status"=FALSE, "code"=0, "source"=""} ("error constant")] -> w37
          tunnel: w36 -> [w45 _]
          event Timeout {
            n142 = event-data() -> ("Time"=w48:u32)  [unwired: 1 in]
            n143 = call <vilib>:"Update Last Execution Time-v2.vi"("Time"=w48, "Helper Loop Periodic Timing in"=w47) -> ("Helper Loop Periodic Timing out"=w46:refnum<class "Helper Loop Periodic Timing.lvclass">)  [unwired: 12 in, 1 out]
            n144 = call <userlib>:"Periodic Trigger__ogtk.vi"("time (ms)"=u32 1000) -> ("Triggered"=w42:bool)  [unwired: 12 in, 2 out]
            n145 = case shown="True" w42 {
              tunnel: w45 -> [_ w51]
              tunnel: [_ w50] -> w44
              frame False {
              }
              frame True {
                n146 = call-poly <vilib>:"Delacor_lib_QMH_Enqueue Message (poly).vi"("Message"="Ping", "Message Queue in"=w51) -> ("error out"=w50:errorcluster)  [unwired: 8 in, 1 out]
              }
            }
          }
          event User Event {
            n147 = event-data() -> ()  [unwired: 1 in, 1 out]
          }
        }
        n148 = call-dynamic "Delacor_lib_QMH_Error Handler - Helper Loop.vi"("Error Debug"=w35, "error in"=w37, "Message Queue in"=w36) -> ()  [unwired: 7 in, 2 out]
      }
      n149 = call <vilib>:"Stop Helper Loop.vi"("Helper Loop Periodic Timing in"=w18) -> ()  [unwired: 1 out]
      n150 = Unregister For Events(event registration refnum=w23) -> ()  [unwired: 1 in, 1 out]
    }
    frame Error {
      # "Synchronize Caller Events.vi will inform Start Module.vi that the module has launched and will let the code calling Start Module.vi register for broadcasts and would permit the caller receive the broadcast that an error occurred at launch time."
      n151 = call-dynamic "Delacor_lib_QMH_Release Message Queue.vi"("error in"=w301, "Message Queue"=w294) -> ("error out"=w300:errorcluster)  [unwired: 9 in]
      n152 = call "Synchronize Caller Events.vi"("Singleton Module Admin in"=w295) -> ("error out"=w302:errorcluster)  [unwired: 9 in, 1 out]
      n153 = call "Module Name--constant.vi"() -> ("Module Name"=w298:string)  [unwired: 11 in]
      n154 = Format Into String(format string="An error occurred during initialization. %s is no longer running.", w298) -> (resulting string=w296:string)  [unwired: 2 in, 1 out]
      n155 = Merge Errors(w300, w302) -> (w303:errorcluster)
      n156 = call "Error Reported.vi"("Additional Information"=w296, "Error"=w303) -> ()  [unwired: 9 in, 1 out]
    }
  }
  n157 = Merge Errors(w14, w17) -> (w13:errorcluster)
  n158 = call "Close Module.vi"("error in"=w13, "Module Admin in"=w8) -> ("error out"=w15:errorcluster, "External Launch"=w2:bool, "Module Admin out"=w3:refnum<class "Delacor_lib_QMH_Module Admin.lvclass">)  [unwired: 7 in]
  n159 = Unregister For Events(event registration refnum=w7, error in=w15) -> (error out=w12:errorcluster)
  "error out" <- w12
  n160 = case "External Launch?" shown="True" w2 {
    tunnel: w12 -> [_ w304]
    frame False {
    }
    frame True {
      n161 = case shown="No Error" w304 {
        frame No Error {
          n162 = invoke on="Invoke Node" class="VI" method="FP.Close"() -> ()  [unwired: 3 in, 3 out]
        }
        frame Error {
          n163 = invoke on="Invoke Node" class="VI" method="FP.Open"("Activate"=TRUE ("Activate?")) -> ()  [unwired: 4 in, 5 out]
        }
      }
    }
  }
  n164 = local write "Module Admin"(w3) -> ()
